vi "Calculate-MSCN cycle index.vi"(9 "Number of pixels in ROI":i32, 11 "Unity based index of miniscan point":i32) -> (2 "MSCN Cycle index (unity based)":i32)   [LabVIEW 2013]
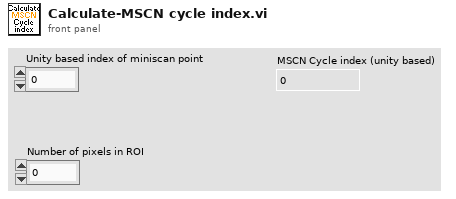
[diagram p1: front panel]
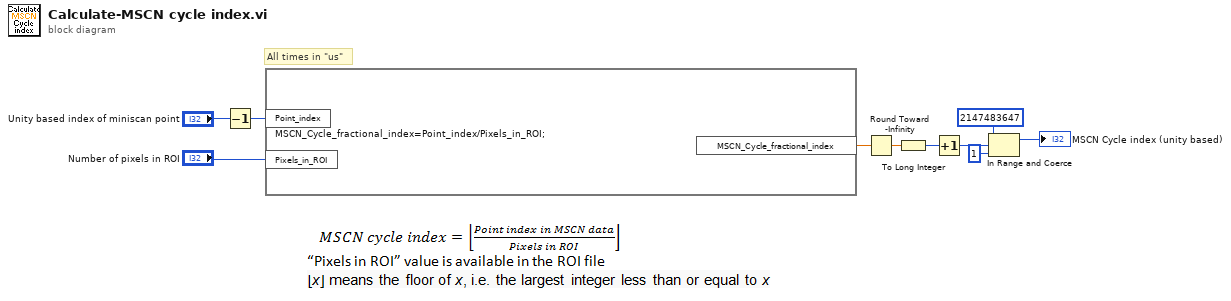
[diagram p0: block diagram]
diagram:
  # "All times in \"us\""
  n1 = Decrement(x="Unity based index of miniscan point") -> (x-1=w6:i32)
  n2 = formula code="MSCN_Cycle_fractional_index=Point_index/Pixels_in_ROI;"("Pixels_in_ROI"="Number of pixels in ROI", "Point_index"=w6) -> ("MSCN_Cycle_fractional_index"=w5:dbl)
  n3 = Round Toward -Infinity(1:w5) -> (0:w9:dbl)
  n4 = To Long Integer(number=w9) -> (32bit integer=w8:i32)
  n5 = Increment(x=w8) -> (x+1=w4:i32)
  n6 = In Range and Coerce(upper limit=2147483647, x=w4, lower limit=1) -> (coerced(x)=→"MSCN Cycle index (unity based)":i32)  [unwired: 1 out]
